vi "HCC Read Network Variables.vi"(8 "error in (no error)":errorcluster, 9 "Current Input":dbl, 10 "Network Var Set":u8, 11 "Network Variable Location":i32) -> (0 "error out":errorcluster, 2 "Dryer":T1 {"Display Data (RLT)"."Current Display" format="%.2f"; "Display Data (RLT)"."Cycle Count Display" format="%04d"; "Appliance Details"."Dryer"."Dryer Initial IMC Data"."Maximum Weight (lbf)" format="%03_6g"; "Appliance Details"."Dryer"."Dryer Initial IMC Data"."Average Weight (lbf)" format="%03_6g"; "Appliance Details"."Dryer"."Dryer Initial IMC Data"."Minimum Weight (lbf)" format="%03_6g"; "Appliance Details"."Dryer"."Dryer Initial IMC Data"."CEF (lbf/kWh)" format="%03_6g"; "Appliance Details"."Dryer"."Dryer Initial IMC Data"."Actual Final RMC (%)" format="%03_6g"; "Appliance Details"."Dryer"."Dryer Initial IMC Data"."Tolerance(%)" format="%0#_6g"; "Appliance Details"."Dryer"."Dryer Initial IMC Data"."Bone Dry Wt(lbs)" format="%03_6g"; "Appliance Details"."Dryer"."Dryer Initial IMC Data"."RMC (Desired %)" format="%0#_6g"; "Appliance Details"."Dryer"."Dryer Initial IMC Data"."Actual Initial RMC (%)" format="%03_6g"; "Appliance Details"."Dryer"."Dryer Initial IMC Data"."Measured IMC (lbs)" format="%0#_6g"}, 5 "Current Output":dbl)   [LabVIEW 2016]
uses:
  Utility/Save File/Public/Type Definitions/Save File Washer.ctl
  Utility/Save File/File Setup (Public)/Type Definition/Save File DISH Dishwasher Details.ctl
  <vilib>/Platform/fileVersionInfo.llb/FileVersionInformation.ctl
  Washer DOE/Type Definitions/DOE Appliance Common.ctl
  Utility/Custom Pallet Controls/Custom Pallet String.ctl
  Utility/Save File/File Setup (Public)/Type Definition/DPT IMC Data.ctl
  Washer DOE/Type Definitions/DOE Dryer Standard.ctl
  Utility/Save File/Public/Type Definitions/Save File Appliance Display.ctl
  Utility/Save File/Public/Type Definitions/Save File Unit Type.ctl
  Utility/Save File/Save File.lvlib
  Utility/Save File/File Setup.lvlib
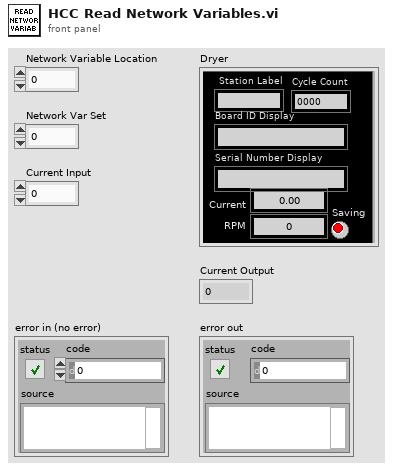
[diagram p1: front panel]
types:
  T1 = typedef "Save File.lvlib/Save File Washer.ctl" = cluster{"Appliance Details":T2, "Display Data (RLT)":T8}
  T2 = typedef "File Setup.lvlib/Save File DISH Dishwasher Details.ctl" = cluster{"FileVersionInfo":T3, "Dishwasher Info":cluster{"Open Cup Weight (gm):":dbl, "Auto Cup Weight (gm):":dbl, "Detergent-Dish:":string, "Inlet Temperature-Dish:":string, "Cycle Mode-Dish:":string, "Unit Control-Dish:":string, "Manufacturer-Dish:":string}, "Washer Info":cluster{"Hot Water Temperature (Fahrenheit):":string, "Cold Water Temperature (Fahrenheit):":string, "Capacity (cu.ft):":dbl, "Initial Cloth Weight:":dbl, "Cloth Lot:":i32, "Model Family:":string, "Program Name:":string, "Cycle Selection:":string, "Wash Temperature:":string, "Rinse Temperature:":string, "Load Size:":string}, "File Name Output Array":string[][], "Calibration Output Array":string[][], "Appliance Common":T4, "Water Heater":cluster{"Heating Mode:":string}, "Dryer":cluster{"Heat Setting:":T5, "Washer Water Temperature (60 ± 5°F):":u16, "Water Hardness (PPM):":u16, "Dryness Setting:":T5, "Dryer Type:":string, "Exhaust:":string, "Drying Cycle:":string, "Load Type:":string, "Nominal Load Weight":string, "Dryer Initial IMC Data":T6}}
  T3 = typedef "FileVersionInformation.ctl" = cluster{"FileVersion":string, "ProductName":string, "InternalName":string, "CompanyName":string, "LegalCopyright":string, "FileDescription":string}
  T4 = typedef "DOE Appliance Common.ctl" = cluster{"Engineer:":string, "Model Number:":string, "Serial Number:":string, "Comments:":string, "Station ID:":string, "Technician:":string, "TR Number:":string, "Lab ID:":string, "Voltage:":string, "Water Pressure (PSI):":string, "Test Date:":string, "Computer Name:":string, "IP Address:":string, "Ambient RH:":string, "Frequency:":string, "Build:":string, "Filename:":string, "Test Type:":string, "Load Run #:":i32, "Ambient Temperature (F):":string, "File Path:":path, "Cycles Per Year":u32}
  T5 = typedef "Custom Pallet String.ctl" = string
  T6 = typedef "DPT IMC Data.ctl" = cluster{"Measured IMC (lbs)":dbl, "Actual Initial RMC (%)":dbl, "RMC (Desired %)":dbl, "Bone Dry Wt(lbs)":dbl, "Tolerance(%)":dbl, "Actual Final RMC (%)":dbl, "CEF (lbf/kWh)":dbl, "Minimum Weight (lbf)":dbl, "Average Weight (lbf)":dbl, "Maximum Weight (lbf)":dbl, "Measured IMC In Range?":bool, "Moisture Reduction Factor":dbl, "Field Use Factor":dbl, "Empty Dryer Cold Weigth":dbl, "Energy Standard":T7, "Weight Cloth (lbs)":dbl, "Relative Moisture Content (%)":dbl, "Relative Moisture Content - Avg (%)":dbl}
  T7 = typedef "DOE Dryer Standard.ctl" = enum16{"D2-Automatic Dryer", "D2-Timer Dryer", "D1-Automatic Dryer", "D1-Timer Dryer", "Other"}
  T8 = typedef "Save File Appliance Display.ctl" = cluster{"Status Color":u32, "Serial Number Display":string, "Cycle Count Display":i32, "Station Label Display":string, "Current Run Start Time Display":dbl, "Board ID Display":string, "RPM Display":u32, "Current Display":dbl, "Current Path Display":path, "Saving Display":bool, "Unit Type Display":T9, "Total Time On Display":dbl, "UI Button":bool}
  T9 = typedef "Save File.lvlib/Save File Unit Type.ctl" = enum32{"", "Viper", "Hawk", "2015"}
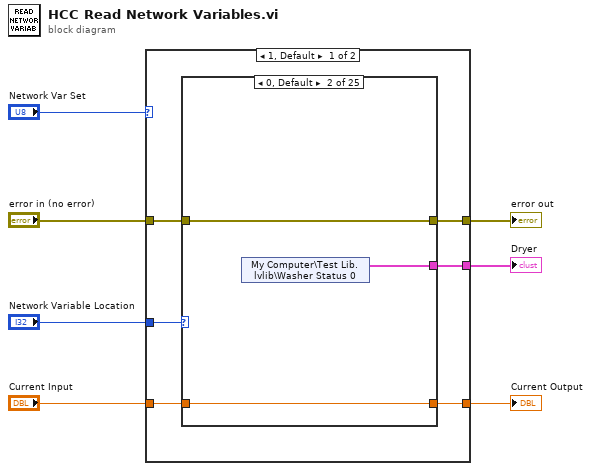
[diagram p0: block diagram]
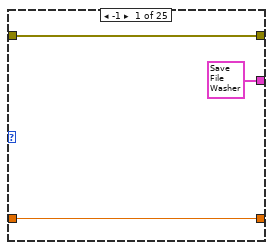
[diagram p2: hidden frame]
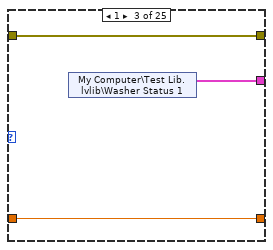
[diagram p3: hidden frame]
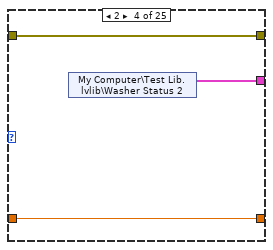
[diagram p4: hidden frame]
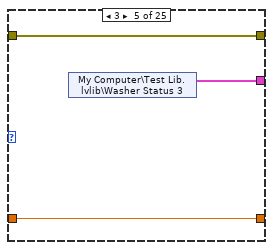
[diagram p5: hidden frame]
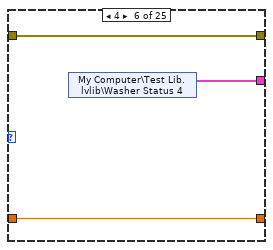
[diagram p6: hidden frame]
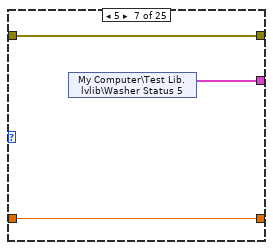
[diagram p7: hidden frame]
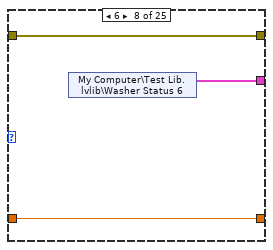
[diagram p8: hidden frame]
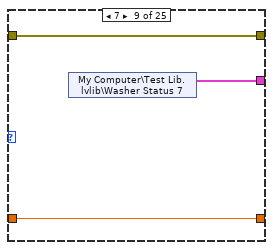
[diagram p9: hidden frame]
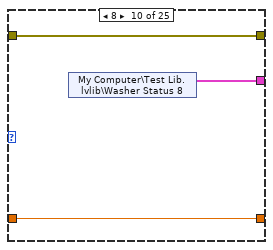
[diagram p10: hidden frame]
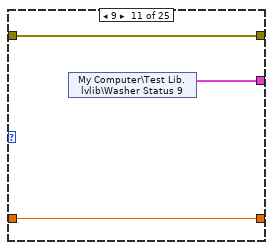
[diagram p11: hidden frame]
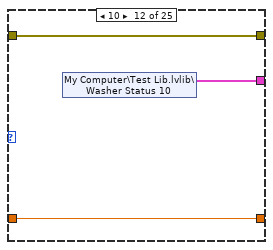
[diagram p12: hidden frame]
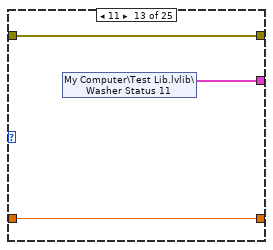
[diagram p13: hidden frame]
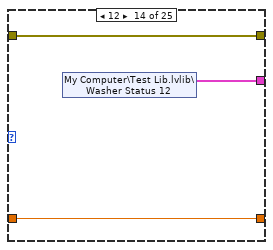
[diagram p14: hidden frame]
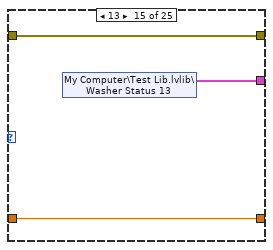
[diagram p15: hidden frame]
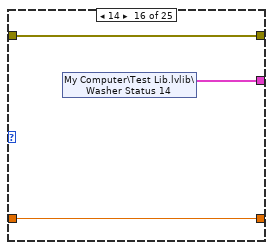
[diagram p16: hidden frame]
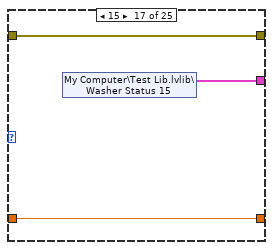
[diagram p17: hidden frame]
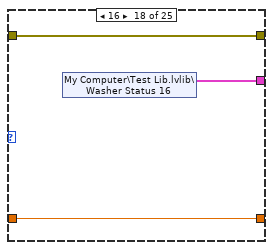
[diagram p18: hidden frame]
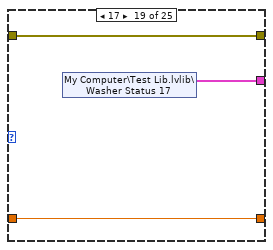
[diagram p19: hidden frame]
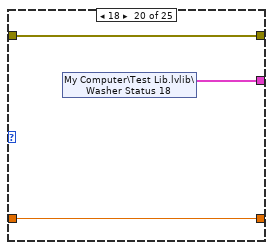
[diagram p20: hidden frame]
diagram:
  n1 = case shown="1, Default" "Network Var Set" {
    tunnel: "Network Variable Location" -> [w13 w92]
    tunnel: [w12 w91] -> w6
    tunnel: [w11 w93] -> w5
    tunnel: "error in (no error)" -> [w10 w94]
    tunnel: [w9 w89] -> w3
    tunnel: "Current Input" -> [w8 w90]
    frame 1, Default {
      n2 = case shown="0, Default" w13 {
        tunnel: [T1 {"Appliance Details"={"FileVersionInfo"={"FileVersion"="", "ProductName"="", "InternalName"="", "CompanyName"="", "LegalCopyright"="", "FileDescription"=""}, "Dishwasher Info"={"Open Cup Weight (gm):"=0.0, "Auto Cup Weight (gm):"=0.0, "Detergent-Dish:"="", "Inlet Temperature-Dish:"="", "Cycle Mode-Dish:"="", "Unit Control-Dish:"="", "Manufacturer-Dish:"=""}, "Washer Info"={"Hot Water Temperature (Fahrenheit):"="", "Cold Water Temperature (Fahrenheit):"="", "Capacity (cu.ft):"=0.0, "Initial Cloth Weight:"=0.0, "Cloth Lot:"=0, "Model Family:"="", "Program Name:"="", "Cycle Selection:"="", "Wash Temperature:"="", "Rinse Temperature:"="", "Load Size:"=""}, "File Name Output Array"=[], "Calibration Output Array"=[], "Appliance Common"={"Engineer:"="", "Model Number:"="", "Serial Number:"="", "Comments:"="", "Station ID:"="", "Technician:"="", "TR Number:"="", "Lab ID:"="", "Voltage:"="", "Water Pressure (PSI):"="", "Test Date:"="", "Computer Name:"="", "IP Address:"="", "Ambient RH:"="", "Frequency:"="", "Build:"="", "Filename:"="", "Test Type:"="", "Load Run #:"=0, "Ambient Temperature (F):"="", "File Path:"=path "", "Cycles Per Year"=60}, "Water Heater"={"Heating Mode:"=""}, "Dryer"={"Heat Setting:"="", "Washer Water Temperature (60 ± 5°F):"=60, "Water Hardness (PPM):"=17, "Dryness Setting:"="", "Dryer Type:"="", "Exhaust:"="", "Drying Cycle:"="", "Load Type:"="", "Nominal Load Weight"="", "Dryer Initial IMC Data"={"Measured IMC (lbs)"=7.0, "Actual Initial RMC (%)"=7.0, "RMC (Desired %)"=100.0, "Bone Dry Wt(lbs)"=7.0, "Tolerance(%)"=5.0, "Actual Final RMC (%)"=7.0, "CEF (lbf/kWh)"=0.0, "Minimum Weight (lbf)"=0.0, "Average Weight (lbf)"=0.0, "Maximum Weight (lbf)"=0.0, "Measured IMC In Range?"=FALSE, "Moisture Reduction Factor"=55.5, "Field Use Factor"=1.04, "Empty Dryer Cold Weigth"=0.0, "Energy Standard"=enum."D2-Automatic Dryer", "Weight Cloth (lbs)"=0.0, "Relative Moisture Content (%)"=0.0, "Relative Moisture Content - Avg (%)"=0.0}}}, "Display Data (RLT)"={"Status Color"=0, "Serial Number Display"="", "Cycle Count Display"=0, "Station Label Display"="", "Current Run Start Time Display"=0.0, "Board ID Display"="", "RPM Display"=0, "Current Display"=0.0, "Current Path Display"=path "", "Saving Display"=FALSE, "Unit Type Display"=enum."", "Total Time On Display"=0.0, "UI Button"=FALSE}} ("Dryer") w17 w20 w23 w26 w29 w32 w35 w38 w42 w46 w49 w52 w55 w58 w61 w64 w67 w70 w73 w76 w79 w82 w85 w88] -> w12
        tunnel: [w16 w19 w22 w25 w28 w31 w34 w37 w40 w43 w45 w48 w51 w54 w57 w60 w63 w66 w69 w72 w75 w78 w81 w84 w87] -> w9
        tunnel: w8 -> [w16 w19 w22 w25 w28 w31 w34 w37 w40 w43 w45 w48 w51 w54 w57 w60 w63 w66 w69 w72 w75 w78 w81 w84 w87]
        tunnel: w10 -> [w14 w18 w21 w24 w27 w30 w33 w36 w39 w41 w44 w47 w50 w53 w56 w59 w62 w65 w68 w71 w74 w77 w80 w83 w86]
        tunnel: [w14 w18 w21 w24 w27 w30 w33 w36 w39 w41 w44 w47 w50 w53 w56 w59 w62 w65 w68 w71 w74 w77 w80 w83 w86] -> w11
        frame -1 {
        }
        frame 0, Default {
          n3 = shared-variable "My Computer\\Test Lib.lvlib\\Washer Status 0"() -> (w17:T1)  [unwired: 1 in, 1 out]
        }
        frame 1 {
          n4 = shared-variable "My Computer\\Test Lib.lvlib\\Washer Status 1"() -> (w20:T1)  [unwired: 1 in, 1 out]
        }
        frame 2 {
          n5 = shared-variable "My Computer\\Test Lib.lvlib\\Washer Status 2"() -> (w23:T1)  [unwired: 1 in, 1 out]
        }
        frame 3 {
          n6 = shared-variable "My Computer\\Test Lib.lvlib\\Washer Status 3"() -> (w26:T1)  [unwired: 1 in, 1 out]
        }
        frame 4 {
          n7 = shared-variable "My Computer\\Test Lib.lvlib\\Washer Status 4"() -> (w29:T1)  [unwired: 1 in, 1 out]
        }
        frame 5 {
          n8 = shared-variable "My Computer\\Test Lib.lvlib\\Washer Status 5"() -> (w32:T1)  [unwired: 1 in, 1 out]
        }
        frame 6 {
          n9 = shared-variable "My Computer\\Test Lib.lvlib\\Washer Status 6"() -> (w35:T1)  [unwired: 1 in, 1 out]
        }
        frame 7 {
          n10 = shared-variable "My Computer\\Test Lib.lvlib\\Washer Status 7"() -> (w38:T1)  [unwired: 1 in, 1 out]
        }
        frame 8 {
          n11 = shared-variable "My Computer\\Test Lib.lvlib\\Washer Status 8"() -> (w42:T1)  [unwired: 1 in, 1 out]
        }
        frame 9 {
          n12 = shared-variable "My Computer\\Test Lib.lvlib\\Washer Status 9"() -> (w46:T1)  [unwired: 1 in, 1 out]
        }
        frame 10 {
          n13 = shared-variable "My Computer\\Test Lib.lvlib\\Washer Status 10"() -> (w49:T1)  [unwired: 1 in, 1 out]
        }
        frame 11 {
          n14 = shared-variable "My Computer\\Test Lib.lvlib\\Washer Status 11"() -> (w52:T1)  [unwired: 1 in, 1 out]
        }
        frame 12 {
          n15 = shared-variable "My Computer\\Test Lib.lvlib\\Washer Status 12"() -> (w55:T1)  [unwired: 1 in, 1 out]
        }
        frame 13 {
          n16 = shared-variable "My Computer\\Test Lib.lvlib\\Washer Status 13"() -> (w58:T1)  [unwired: 1 in, 1 out]
        }
        frame 14 {
          n17 = shared-variable "My Computer\\Test Lib.lvlib\\Washer Status 14"() -> (w61:T1)  [unwired: 1 in, 1 out]
        }
        frame 15 {
          n18 = shared-variable "My Computer\\Test Lib.lvlib\\Washer Status 15"() -> (w64:T1)  [unwired: 1 in, 1 out]
        }
        frame 16 {
          n19 = shared-variable "My Computer\\Test Lib.lvlib\\Washer Status 16"() -> (w67:T1)  [unwired: 1 in, 1 out]
        }
        frame 17 {
          n20 = shared-variable "My Computer\\Test Lib.lvlib\\Washer Status 17"() -> (w70:T1)  [unwired: 1 in, 1 out]
        }
        frame 18 {
          n21 = shared-variable "My Computer\\Test Lib.lvlib\\Washer Status 18"() -> (w73:T1)  [unwired: 1 in, 1 out]
        }
        frame 19 {
          n22 = shared-variable "My Computer\\Test Lib.lvlib\\Washer Status 19"() -> (w76:T1)  [unwired: 1 in, 1 out]
        }
        frame 20 {
          n23 = shared-variable "My Computer\\Test Lib.lvlib\\Washer Status 20"() -> (w79:T1)  [unwired: 1 in, 1 out]
        }
        frame 21 {
          n24 = shared-variable "My Computer\\Test Lib.lvlib\\Washer Status 21"() -> (w82:T1)  [unwired: 1 in, 1 out]
        }
        frame 22 {
          n25 = shared-variable "My Computer\\Test Lib.lvlib\\Washer Status 22"() -> (w85:T1)  [unwired: 1 in, 1 out]
        }
        frame 23 {
          n26 = shared-variable "My Computer\\Test Lib.lvlib\\Washer Status 23"() -> (w88:T1)  [unwired: 1 in, 1 out]
        }
      }
    }
    frame 2 {
      n27 = case shown="0, Default" w92 {
        tunnel: [T1 {"Appliance Details"={"FileVersionInfo"={"FileVersion"="", "ProductName"="", "InternalName"="", "CompanyName"="", "LegalCopyright"="", "FileDescription"=""}, "Dishwasher Info"={"Open Cup Weight (gm):"=0.0, "Auto Cup Weight (gm):"=0.0, "Detergent-Dish:"="", "Inlet Temperature-Dish:"="", "Cycle Mode-Dish:"="", "Unit Control-Dish:"="", "Manufacturer-Dish:"=""}, "Washer Info"={"Hot Water Temperature (Fahrenheit):"="", "Cold Water Temperature (Fahrenheit):"="", "Capacity (cu.ft):"=0.0, "Initial Cloth Weight:"=0.0, "Cloth Lot:"=0, "Model Family:"="", "Program Name:"="", "Cycle Selection:"="", "Wash Temperature:"="", "Rinse Temperature:"="", "Load Size:"=""}, "File Name Output Array"=[], "Calibration Output Array"=[], "Appliance Common"={"Engineer:"="", "Model Number:"="", "Serial Number:"="", "Comments:"="", "Station ID:"="", "Technician:"="", "TR Number:"="", "Lab ID:"="", "Voltage:"="", "Water Pressure (PSI):"="", "Test Date:"="", "Computer Name:"="", "IP Address:"="", "Ambient RH:"="", "Frequency:"="", "Build:"="", "Filename:"="", "Test Type:"="", "Load Run #:"=0, "Ambient Temperature (F):"="", "File Path:"=path "", "Cycles Per Year"=60}, "Water Heater"={"Heating Mode:"=""}, "Dryer"={"Heat Setting:"="", "Washer Water Temperature (60 ± 5°F):"=60, "Water Hardness (PPM):"=17, "Dryness Setting:"="", "Dryer Type:"="", "Exhaust:"="", "Drying Cycle:"="", "Load Type:"="", "Nominal Load Weight"="", "Dryer Initial IMC Data"={"Measured IMC (lbs)"=7.0, "Actual Initial RMC (%)"=7.0, "RMC (Desired %)"=100.0, "Bone Dry Wt(lbs)"=7.0, "Tolerance(%)"=5.0, "Actual Final RMC (%)"=7.0, "CEF (lbf/kWh)"=0.0, "Minimum Weight (lbf)"=0.0, "Average Weight (lbf)"=0.0, "Maximum Weight (lbf)"=0.0, "Measured IMC In Range?"=FALSE, "Moisture Reduction Factor"=55.5, "Field Use Factor"=1.04, "Empty Dryer Cold Weigth"=0.0, "Energy Standard"=enum."D2-Automatic Dryer", "Weight Cloth (lbs)"=0.0, "Relative Moisture Content (%)"=0.0, "Relative Moisture Content - Avg (%)"=0.0}}}, "Display Data (RLT)"={"Status Color"=0, "Serial Number Display"="", "Cycle Count Display"=0, "Station Label Display"="", "Current Run Start Time Display"=0.0, "Board ID Display"="", "RPM Display"=0, "Current Display"=0.0, "Current Path Display"=path "", "Saving Display"=FALSE, "Unit Type Display"=enum."", "Total Time On Display"=0.0, "UI Button"=FALSE}} ("Dryer") w98 w101 w104 w107 w110 w113 w116 w119 w122 w125 w128 w131 w134 w137 w140 w143 w146 w149 w152 w155 w158 w161 w164 w167] -> w91
        tunnel: [w97 w100 w103 w106 w109 w112 w115 w118 w121 w124 w127 w130 w133 w136 w139 w142 w145 w148 w151 w154 w157 w160 w163 w166 w169] -> w89
        tunnel: w90 -> [w97 w100 w103 w106 w109 w112 w115 w118 w121 w124 w127 w130 w133 w136 w139 w142 w145 w148 w151 w154 w157 w160 w163 w166 w169]
        tunnel: w94 -> [w95 w99 w102 w105 w108 w111 w114 w117 w120 w123 w126 w129 w132 w135 w138 w141 w144 w147 w150 w153 w156 w159 w162 w165 w168]
        tunnel: [w95 w99 w102 w105 w108 w111 w114 w117 w120 w123 w126 w129 w132 w135 w138 w141 w144 w147 w150 w153 w156 w159 w162 w165 w168] -> w93
        frame -1 {
        }
        frame 0, Default {
          n28 = shared-variable "My Computer\\Test Lib.lvlib\\Washer Status 24"() -> (w98:T1)  [unwired: 1 in, 1 out]
        }
        frame 1 {
          n29 = shared-variable "My Computer\\Test Lib.lvlib\\Washer Status 25"() -> (w101:T1)  [unwired: 1 in, 1 out]
        }
        frame 2 {
          n30 = shared-variable "My Computer\\Test Lib.lvlib\\Washer Status 26"() -> (w104:T1)  [unwired: 1 in, 1 out]
        }
        frame 3 {
          n31 = shared-variable "My Computer\\Test Lib.lvlib\\Washer Status 27"() -> (w107:T1)  [unwired: 1 in, 1 out]
        }
        frame 4 {
          n32 = shared-variable "My Computer\\Test Lib.lvlib\\Washer Status 28"() -> (w110:T1)  [unwired: 1 in, 1 out]
        }
        frame 5 {
          n33 = shared-variable "My Computer\\Test Lib.lvlib\\Washer Status 29"() -> (w113:T1)  [unwired: 1 in, 1 out]
        }
        frame 6 {
          n34 = shared-variable "My Computer\\Test Lib.lvlib\\Washer Status 30"() -> (w116:T1)  [unwired: 1 in, 1 out]
        }
        frame 7 {
          n35 = shared-variable "My Computer\\Test Lib.lvlib\\Washer Status 31"() -> (w119:T1)  [unwired: 1 in, 1 out]
        }
        frame 8 {
          n36 = shared-variable "My Computer\\Test Lib.lvlib\\Washer Status 32"() -> (w122:T1)  [unwired: 1 in, 1 out]
        }
        frame 9 {
          n37 = shared-variable "My Computer\\Test Lib.lvlib\\Washer Status 33"() -> (w125:T1)  [unwired: 1 in, 1 out]
        }
        frame 10 {
          n38 = shared-variable "My Computer\\Test Lib.lvlib\\Washer Status 34"() -> (w128:T1)  [unwired: 1 in, 1 out]
        }
        frame 11 {
          n39 = shared-variable "My Computer\\Test Lib.lvlib\\Washer Status 35"() -> (w131:T1)  [unwired: 1 in, 1 out]
        }
        frame 12 {
          n40 = shared-variable "My Computer\\Test Lib.lvlib\\Washer Status 36"() -> (w134:T1)  [unwired: 1 in, 1 out]
        }
        frame 13 {
          n41 = shared-variable "My Computer\\Test Lib.lvlib\\Washer Status 37"() -> (w137:T1)  [unwired: 1 in, 1 out]
        }
        frame 14 {
          n42 = shared-variable "My Computer\\Test Lib.lvlib\\Washer Status 38"() -> (w140:T1)  [unwired: 1 in, 1 out]
        }
        frame 15 {
          n43 = shared-variable "My Computer\\Test Lib.lvlib\\Washer Status 39"() -> (w143:T1)  [unwired: 1 in, 1 out]
        }
        frame 16 {
          n44 = shared-variable "My Computer\\Test Lib.lvlib\\Washer Status 40"() -> (w146:T1)  [unwired: 1 in, 1 out]
        }
        frame 17 {
          n45 = shared-variable "My Computer\\Test Lib.lvlib\\Washer Status 41"() -> (w149:T1)  [unwired: 1 in, 1 out]
        }
        frame 18 {
          n46 = shared-variable "My Computer\\Test Lib.lvlib\\Washer Status 42"() -> (w152:T1)  [unwired: 1 in, 1 out]
        }
        frame 19 {
          n47 = shared-variable "My Computer\\Test Lib.lvlib\\Washer Status 43"() -> (w155:T1)  [unwired: 1 in, 1 out]
        }
        frame 20 {
          n48 = shared-variable "My Computer\\Test Lib.lvlib\\Washer Status 44"() -> (w158:T1)  [unwired: 1 in, 1 out]
        }
        frame 21 {
          n49 = shared-variable "My Computer\\Test Lib.lvlib\\Washer Status 45"() -> (w161:T1)  [unwired: 1 in, 1 out]
        }
        frame 22 {
          n50 = shared-variable "My Computer\\Test Lib.lvlib\\Washer Status 46"() -> (w164:T1)  [unwired: 1 in, 1 out]
        }
        frame 23 {
          n51 = shared-variable "My Computer\\Test Lib.lvlib\\Washer Status 47"() -> (w167:T1)  [unwired: 1 in, 1 out]
        }
      }
    }
  }
  "Dryer" <- w6
  "error out" <- w5
  "Current Output" <- w3
